vi "Disconnect.vi"(8 "error in (no error)":errorcluster, 11 "GRPCClient in":refnum<class "GRPCClient.lvclass">) -> (0 "error out":errorcluster, 3 "GRPCClient out":refnum<class "GRPCClient.lvclass">)   [LabVIEW 2019, in "GRPCClient.lvclass"]
uses:
  GRPCClient.lvclass
  GRPCClient.lvclass/GRPCClient.ctl
  Autogenerated/Micron_client/Micron_client.lvlib
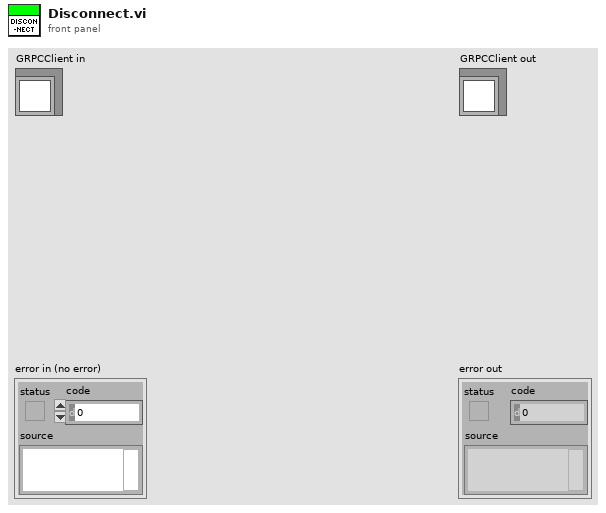
[diagram p1: front panel]
types:
  T1 = typedef "grpc-lvsupport-release.lvlib/grpcId.ctl" = u64
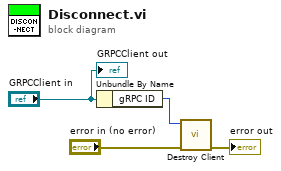
[diagram p0: block diagram]
diagram:
  n1 = Unbundle By Name("GRPCClient in") -> ("gRPC ID"=w1:T1)
  n2 = call "Destroy Client.vi"("error in"="error in (no error)", "gRPC ID"=w1) -> ("error out"=→"error out":errorcluster)  [unwired: 9 in]
  "GRPCClient out" <- "GRPCClient in"
